vi "FTW-CodeGen-Initialize.vi"(5 "XRef":refnum<vi>, 7 "Items":i32=1) -> (4 "State Out":T1 {"Width" format="%dpx"})   [LabVIEW 2015, in "FTW-Dataflow-Burrow.xnode"]
uses:
  FTW-Dataflow-Burrow.xnode
  FTW-CodeGen-State.ctl
panel:
  # "Inputs"
  # "Outputs"
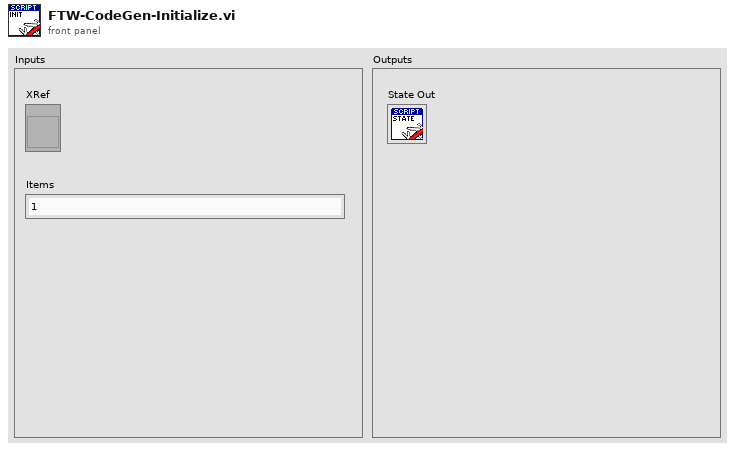
[diagram p1: front panel]
types:
  T1 = typedef "FTW-Dataflow-Burrow.xnode/FTW-CodeGen-State.ctl" = cluster{"InputTerminals":cluster{"Wired?":bool, "ID":string, "DataName":string, "DataColor":u32, "Type":variant}[], "EnableTiming?":bool, "Width":i32}
  T2 = cluster{"Wired?":bool, "ID":string, "DataName":string, "DataColor":u32, "Type":variant}
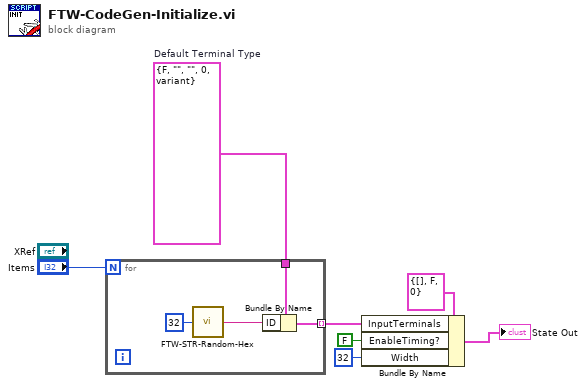
[diagram p0: block diagram]
diagram:
  w3 = T2 {"Wired?"=FALSE, "ID"="", "DataName"="", "DataColor"=0, "Type"=variant(variant variant)}  # Default Terminal Type
  n1 = for {
    N: "Items" -> [_]
    tunnel: [w10] -> w4 mode=indexing
    tunnel: w3 -> [w11]
    n2 = call "FTW-STR-Random-Hex.vi"("String Length"=32) -> ("Random Hex String"=w9:string)  [unwired: 3 in]
    n3 = Bundle By Name(cluster=w11, "ID"=w9) -> (w10:T2)
  }
  n4 = Bundle By Name(cluster=T1 {"InputTerminals"=[], "EnableTiming?"=FALSE, "Width"=0} ("State Out"), "InputTerminals"=w4, "EnableTiming?"=FALSE, "Width"=32) -> (→"State Out":T1)
